vi "Get All Platforms.vi"(8 "error in (no error)":errorcluster, 11 "TargetPluginManager in":refnum<class "PlatformPluginManager.lvclass">) -> (0 "error out":errorcluster, 2 "Platforms":refnum<class "DeployPlatform.lvclass">[](array[class]), 3 "TargetPluginManager out":refnum<class "PlatformPluginManager.lvclass">)   [LabVIEW 2020, in "PicoG-Core.lvlib" / "PlatformPluginManager.lvclass"]
uses:
  PlatformPluginManager.lvclass
  DeployPlatform/DeployPlatform.lvclass
  PlatformPluginManager.lvclass/PlatformPluginManager.ctl
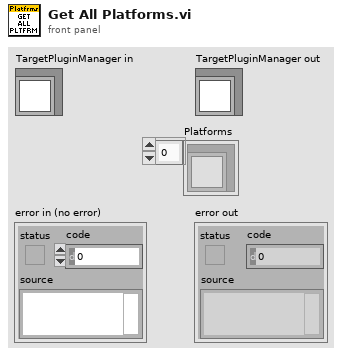
[diagram p1: front panel]
types:
  T1 = typedef "PicoG-Core.lvlib/PlatformPluginManager.lvclass/Ref Data.ctl" = cluster{"Platforms":refnum<class "DeployPlatform.lvclass">[], "Last Platform":refnum<class "DeployPlatform.lvclass">, "Last Resource":refnum<class "DeployResource.lvclass">}
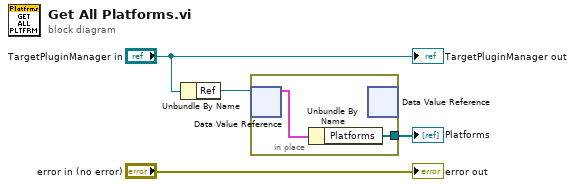
[diagram p0: block diagram]
diagram:
  n1 = Unbundle By Name("TargetPluginManager in") -> ("Ref"=w3:refnum<data-value>)
  n2 = in-place {
    in-place-border: [w5] -> w1
    n3 = in-place-dvr #1(w3) -> (w6:T1)  [unwired: 1 out]
    n4 = Unbundle By Name(w6) -> ("Platforms"=w5:refnum<class "DeployPlatform.lvclass">[])
    n5 = in-place-dvr #1() -> ()  [unwired: 1 in, 2 out]
  }
  "Platforms" <- w1
  "error out" <- "error in (no error)"
  "TargetPluginManager out" <- "TargetPluginManager in"
